vi "ep_Flicker Constants3B.vi"(0 "voltage system":enum16{"120 V", "230 V"}(ring), 5 "input sampling rate":dbl=400.0) -> (3 "A":dbl, 4 "B":dbl, 6 "C":dbl, 8 "D":dbl, 10 "E":dbl, 13 "H":dbl, 14 "G":dbl, 15 "F":dbl)   [LabVIEW 2011, in "NI_EP_Power Quality.lvlib"]
uses:
  <vilib>/addons/Electrical Power/PQ/NI_EP_Power Quality.lvlib
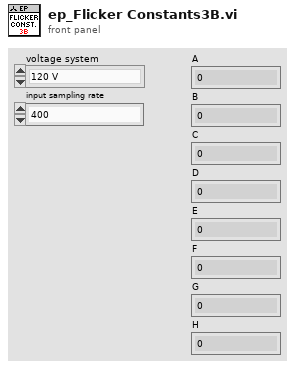
[diagram p1: front panel]
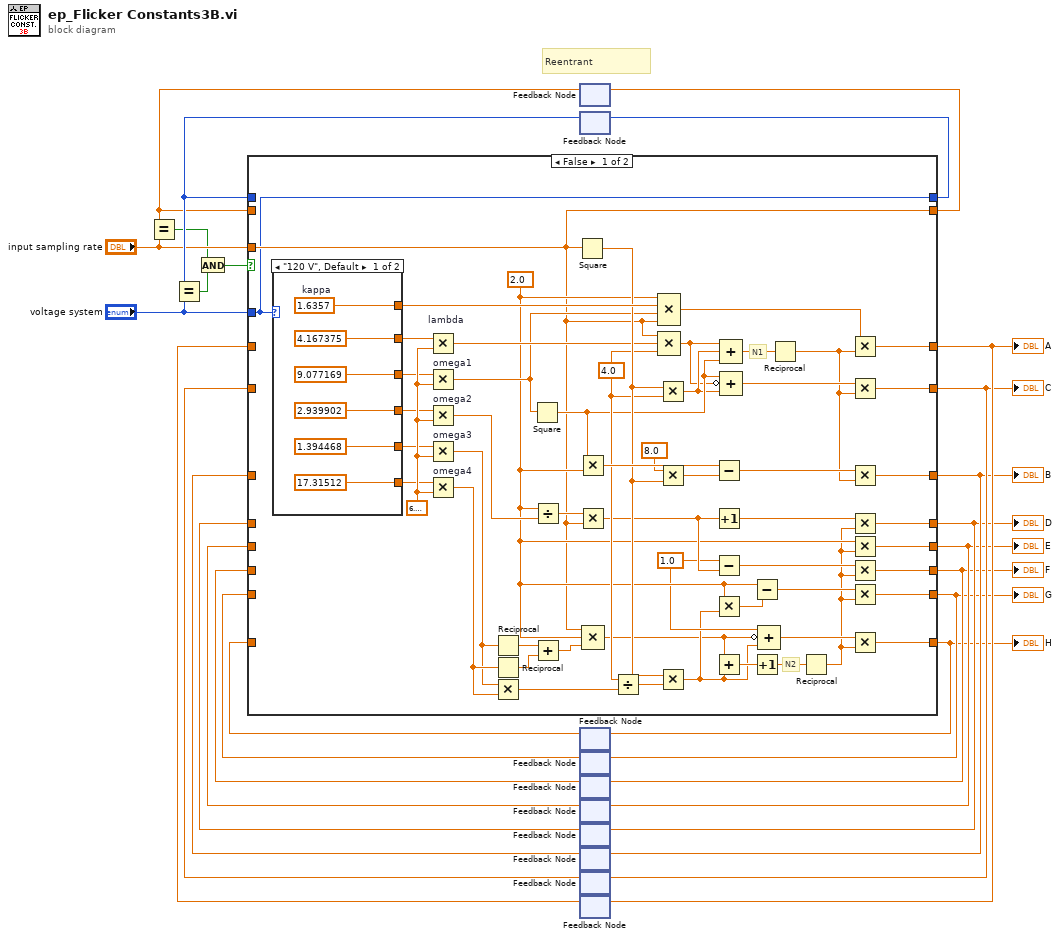
[diagram p0: block diagram]
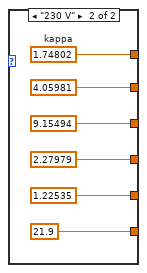
[diagram p2: hidden frame]
diagram:
  # "Reentrant"
  n1 = feedback #1() -> (w6:dbl)  [unwired: 1 in]
  n2 = Equal?(x=w6, y="input sampling rate") -> (x = y?=w3:bool)
  n3 = feedback #2() -> (w8:enum16{"120 V", "230 V"})  [unwired: 1 in]
  n4 = Equal?(x=w8, y="voltage system") -> (x = y?=w5:bool)
  n5 = And(x=w3, y=w5) -> (x .and. y?=w9:bool)
  n6 = feedback #3() -> (w11:dbl)  [unwired: 1 in]
  n7 = feedback #4() -> (w13:dbl)  [unwired: 1 in]
  n8 = feedback #5() -> (w15:dbl)  [unwired: 1 in]
  n9 = feedback #6() -> (w17:dbl)  [unwired: 1 in]
  n10 = feedback #7() -> (w22:dbl)  [unwired: 1 in]
  n11 = feedback #8() -> (w23:dbl)  [unwired: 1 in]
  n12 = feedback #9() -> (w24:dbl)  [unwired: 1 in]
  n13 = feedback #10() -> (w25:dbl)  [unwired: 1 in]
  n14 = case shown="False" w9 {
    tunnel: [w68 w92] -> w21
    tunnel: "voltage system" -> [w26 _]
    tunnel: [w67 w94] -> w19
    tunnel: [w66 w93] -> w20
    tunnel: [w65 w95] -> w18
    tunnel: [w61 w97] -> w14
    tunnel: [w58 w98] -> w12
    tunnel: [w55 w99] -> w10
    tunnel: "input sampling rate" -> [w27 _]
    tunnel: [w29 w96] -> w16
    tunnel: [w27 w100] -> w1
    tunnel: [w26 w101] -> w2
    tunnel: w8 -> [_ w101]
    tunnel: w6 -> [_ w100]
    tunnel: w11 -> [_ w99]
    tunnel: w13 -> [_ w98]
    tunnel: w15 -> [_ w97]
    tunnel: w17 -> [_ w96]
    tunnel: w22 -> [_ w95]
    tunnel: w23 -> [_ w94]
    tunnel: w24 -> [_ w93]
    tunnel: w25 -> [_ w92]
    frame False {
      w33 = 1.0
      w46 = 4.0
      w36 = 2.0
      w79 = 6.283185307179586
      # "N1"
      # "N2"
      n15 = case shown="\"120 V\", Default" w26 {
        tunnel: [4.167375 ("k") 4.05981 ("k")] -> w78
        tunnel: [9.077169 ("k") 9.15494 ("k")] -> w77
        tunnel: [2.939902 ("k") 2.27979 ("k")] -> w76
        tunnel: [1.394468 ("k") 1.22535 ("k")] -> w75
        tunnel: [17.31512 ("k") 21.9 ("k")] -> w74
        tunnel: [w85 w91] -> w53
        frame "120 V", Default {
          w85 = 1.6357  # kappa
        }
        frame "230 V" {
          w91 = 1.74802  # kappa
        }
      }
      n16 = Multiply "lambda"(x=w78, y=w79) -> (x*y=w47:dbl)
      n17 = Multiply "omega1"(x=w77, y=w79) -> (x*y=w45:dbl)
      n18 = Multiply "omega2"(x=w76, y=w79) -> (x*y=w63:dbl)
      n19 = Multiply "omega3"(x=w75, y=w79) -> (x*y=w56:dbl)
      n20 = Multiply "omega4"(x=w74, y=w79) -> (x*y=w57:dbl)
      n21 = Reciprocal(x=w56) -> (1/x=w72:dbl)
      n22 = Reciprocal(x=w57) -> (1/x=w73:dbl)
      n23 = Multiply(x=w56, y=w57) -> (x*y=w49:dbl)
      n24 = Square(x=w45) -> (x^2=w43:dbl)
      n25 = Divide(x=w36, y=w63) -> (x/y=w62:dbl)
      n26 = Add(x=w72, y=w73) -> (x+y=w54:dbl)
      n27 = Square(x=w27) -> (x^2=w48:dbl)
      n28 = Multiply(x=w43, y=w36) -> (x*y=w71:dbl)
      n29 = Multiply(x=w62, y=w27) -> (x*y=w39:dbl)
      n30 = Compound Arithmetic op=MULTIPLY(w27, w36, w54) -> (w28:dbl)
      n31 = Divide(x=w46, y=w49) -> (x/y=w51:dbl)
      n32 = Compound Arithmetic op=MULTIPLY(w36, w53, w45, w27) -> (w52:dbl)
      n33 = Compound Arithmetic op=MULTIPLY(w27, w47, w46) -> (w40:dbl)
      n34 = Multiply(x=w48, y=w46) -> (x*y=w42:dbl)
      n35 = Multiply(x=8.0, y=w48) -> (x*y=w70:dbl)
      n36 = Multiply(x=w48, y=w51) -> (x*y=w32:dbl)
      n37 = Subtract(x=w71, y=w70) -> (x-y=w69:dbl)
      n38 = Increment(x=w39) -> (x+1=w38:dbl)
      n39 = Subtract(x=w33, y=w39) -> (x-y=w64:dbl)
      n40 = Multiply(x=w36, y=w32) -> (x*y=w59:dbl)
      n41 = Add(x=w28, y=w32) -> (x+y=w37:dbl)
      n42 = Compound Arithmetic op=ADD(w40, w42, w43) -> (w44:dbl)
      n43 = Compound Arithmetic op=ADD(w43, invert w40, w42) -> (w41:dbl)
      n44 = Subtract(x=w36, y=w59) -> (x-y=w60:dbl)
      n45 = Increment(x=w37) -> (x+1=w35:dbl)
      n46 = Compound Arithmetic op=ADD(w33, invert w28, w32) -> (w31:dbl)
      n47 = Reciprocal(x=w44) -> (1/x=w34:dbl)
      n48 = Reciprocal(x=w35) -> (1/x=w30:dbl)
      n49 = Multiply(x=w52, y=w34) -> (x*y=w68:dbl)
      n50 = Multiply(x=w41, y=w34) -> (x*y=w66:dbl)
      n51 = Multiply(x=w69, y=w34) -> (x*y=w67:dbl)
      n52 = Multiply(x=w38, y=w30) -> (x*y=w65:dbl)
      n53 = Multiply(x=w36, y=w30) -> (x*y=w29:dbl)
      n54 = Multiply(x=w64, y=w30) -> (x*y=w61:dbl)
      n55 = Multiply(x=w60, y=w30) -> (x*y=w58:dbl)
      n56 = Multiply(x=w31, y=w30) -> (x*y=w55:dbl)
    }
    frame True {
    }
  }
  "A" <- w21
  "B" <- w19
  "C" <- w20
  "D" <- w18
  "E" <- w16
  "F" <- w14
  "G" <- w12
  "H" <- w10
  n57 = feedback-in #1(w1) -> ()
  n58 = feedback-in #2(w2) -> ()
  n59 = feedback-in #3(w10) -> ()
  n60 = feedback-in #4(w12) -> ()
  n61 = feedback-in #5(w14) -> ()
  n62 = feedback-in #6(w16) -> ()
  n63 = feedback-in #7(w18) -> ()
  n64 = feedback-in #8(w19) -> ()
  n65 = feedback-in #9(w20) -> ()
  n66 = feedback-in #10(w21) -> ()
